vi "Convert Boolean to DBL Array.vi"(11 "Boolean":bool) -> (3 "DBL Array":dbl[](array[numeric]))   [LabVIEW 2013, in "Diagnostics Addon Engine.lvlib"]
uses:
  Diagnostics Addon Engine.lvlib
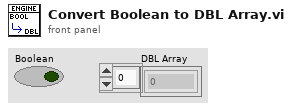
[diagram p1: front panel]
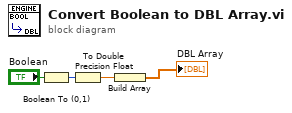
[diagram p0: block diagram]
diagram:
  n1 = Boolean To (0,1)(Boolean="Boolean") -> (0, 1=w2:i16)
  n2 = To Double Precision Float(number=w2) -> (double precision float=w3:dbl)
  n3 = Build Array(w3) -> (→"DBL Array":dbl[])
